vi "Read B.vi"(8 "error in (no error)":errorcluster, 11 "Subtract in":refnum<class "Subtract.lvclass">) -> (0 "error out":errorcluster, 2 "B":dbl, 3 "Subtract out":refnum<class "Subtract.lvclass">)   [LabVIEW 2023, in "Subtract.lvclass"]
uses:
  Subtract.lvclass
  Subtract.lvclass/Subtract.ctl
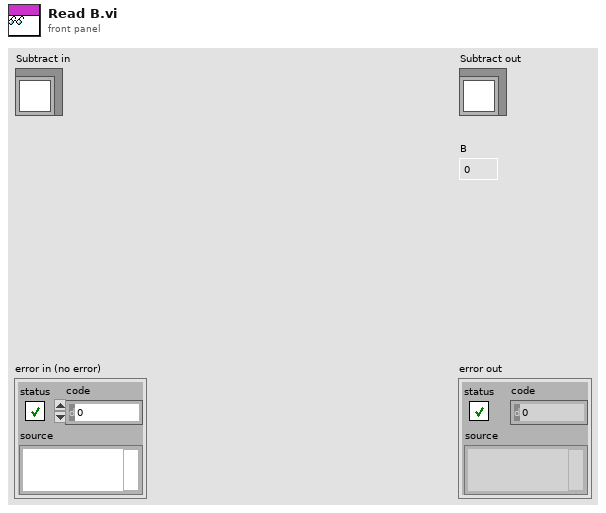
[diagram p1: front panel]
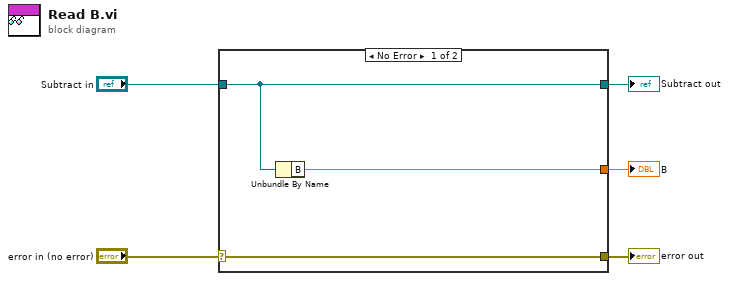
[diagram p0: block diagram]
diagram:
  n1 = case shown="No Error" "error in (no error)" {
    selector: "error in (no error)" -> [w8 w9]
    tunnel: [w8 w9] -> w4
    tunnel: [w7 w10] -> w2
    tunnel: "Subtract in" -> [w7 w10]
    tunnel: [w6 _] -> w1
    frame No Error {
      n2 = Unbundle By Name(w7) -> ("B"=w6:dbl)
    }
    frame Error {
    }
  }
  "error out" <- w4
  "Subtract out" <- w2
  "B" <- w1
